vi "Find Tests.vi"(8 "error in (no error)":errorcluster, 10 "Project Refnum":refnum<vi>, 11 "LVUnit Test Discoverer in":refnum<class "LVUnit Test Discoverer.lvclass">) -> (0 "error out":errorcluster, 2 "Test Cases":refnum<class "Test Case.lvclass">[](array[class]), 3 "LVUnit Test Discoverer out":refnum<class "LVUnit Test Discoverer.lvclass">)   [LabVIEW 2017, in "LVUnit Test Discoverer.lvclass"]
doc: "Finds the tests available from the specified project refnum."
uses:
  LVUnit Test Discoverer.lvclass
  Test Case/Test Case.lvclass
  Json Data Reader/Json Data Reader.lvclass
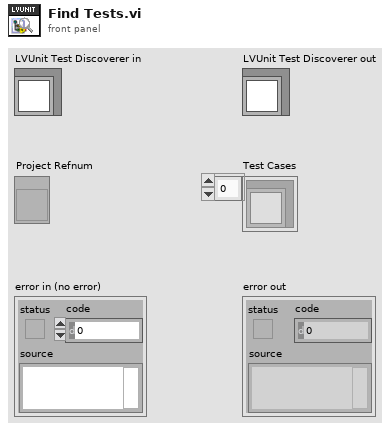
[diagram p1: front panel]
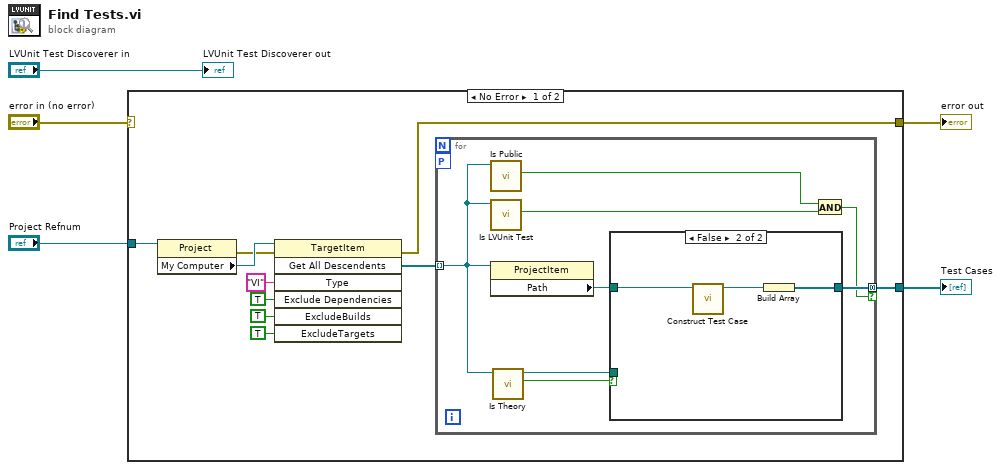
[diagram p0: block diagram]
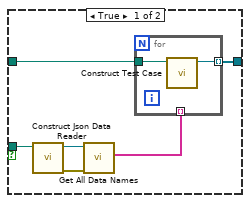
[diagram p2: hidden frame]
diagram:
  n1 = case shown="No Error" "error in (no error)" {
    selector: "error in (no error)" -> [_ w35]
    tunnel: "Project Refnum" -> [w15 _]
    tunnel: [w11 _] -> w3
    tunnel: [w8 w35] -> w2
    frame No Error {
      n2 = property class="Project"(reference=w15) -> (error out=w9:errorcluster, "My Computer"=w14:refnum<vi>)  [unwired: 1 in, 1 out]
      n3 = invoke class="TargetItem" method="Get All Descendents"(reference=w14, error in=w9, "Type"="VI", "Exclude Dependencies"=TRUE ("ExcludeDependencies"), "ExcludeBuilds"=TRUE, "ExcludeTargets"=TRUE) -> (error out=w8:errorcluster, "All Descendents"=w12:refnum<vi>[])  [unwired: 1 in, 5 out]
      n4 = for {
        tunnel: w12 -> [w19] mode=indexing
        tunnel: [w23] -> w11 mode=concatenating if=w16
        workers-P: _ -> [_]
        n5 = call "Is Public.vi"("ProjectItem Refnum"=w19) -> ("Is Private"=w17:bool)  [unwired: 10 in]
        n6 = call "Is LVUnit Test.vi"("ProjectItem Refnum"=w19) -> ("Is LVUnit Test"=w18:bool)  [unwired: 10 in]
        n7 = property class="ProjectItem"(reference=w19) -> ("Path"=w22:path)  [unwired: 1 in, 2 out]
        n8 = call "Is Theory.vi"("ProjectItem Refnum"=w19) -> ("Is Theory"=w20:bool, "Json File"=w21:path)  [unwired: 9 in]
        n9 = case shown="False" w20 {
          tunnel: [w29 w32] -> w23
          tunnel: w22 -> [w28 w33]
          tunnel: w21 -> [w27 _]
          frame True {
            n10 = call "Construct Json Data Reader.vi"("Json File"=w27) -> ("error out"=w25:errorcluster, "Json Data Reader"=w26:refnum<class "Json Data Reader.lvclass">)  [unwired: 9 in]
            n11 = call "Get All Data Names.vi"("error in (no error)"=w25, "Json Data Reader in"=w26) -> ("Data Names"=w24:string[])  [unwired: 7 in, 2 out]
            n12 = for {
              tunnel: [w31] -> w29 mode=indexing
              tunnel: w28 -> [w30]
              tunnel: w24 -> [_] mode=indexing
              n13 = call "Construct Test Case.vi"("Path"=w30) -> ("Test Case"=w31:refnum<class "Test Case.lvclass">)  [unwired: 9 in, 1 out]
            }
          }
          frame False {
            n14 = call "Construct Test Case.vi"("Path"=w33) -> ("Test Case"=w34:refnum<class "Test Case.lvclass">)  [unwired: 9 in, 1 out]
            n15 = Build Array(w34) -> (w32:refnum<class "Test Case.lvclass">[])
          }
        }
        n16 = And(x=w17, y=w18) -> (x .and. y?=w16:bool)
      }
    }
    frame Error {
    }
  }
  "error out" <- w2
  "Test Cases" <- w3
  "LVUnit Test Discoverer out" <- "LVUnit Test Discoverer in"
